vi "Subtract XY (multiple).vi"(8 "error in (no error)":errorcluster, 9 "y":cluster{"X-array":dbl[], "Y-array":dbl[]}, 10 "x":cluster{"X-array":dbl[], "Y-array":dbl[]}, 11 "XY-data":cluster{"X-array":dbl[], "Y-array":dbl[]}[](array[cluster]) {"Y-array" format="%.2p"; "X-array" format="%.2p"}) -> (0 "error out":errorcluster, 3 "XY-data out":cluster{"X-array":dbl[], "Y-array":dbl[]}[](array[cluster]) {"Y-array" format="%.2p"; "X-array" format="%.2p"})   [LabVIEW 2016, in "xy_utilities.lvlib"]
doc: "Subtract <b>x</b>'s x array from the x array of <b>XY-data</b>\nSubtract <b>y</b>'s y array from the y array of <b>XY-data</b>\n\nWire data to the data input to determine the polymorphic instance to use or manually select the instance."
uses:
  xy_utilities.lvlib
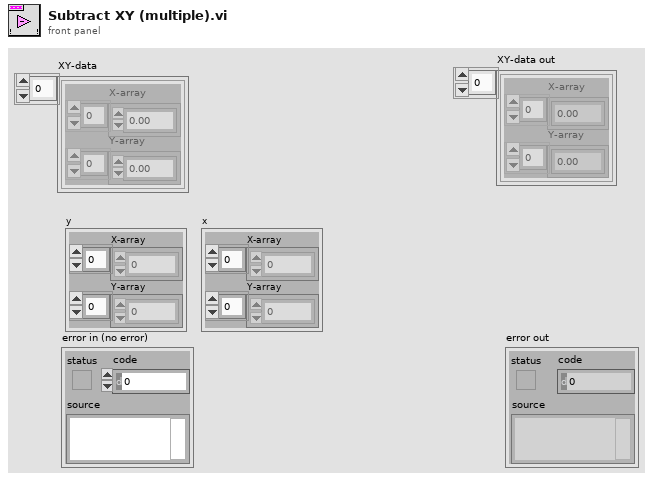
[diagram p1: front panel]
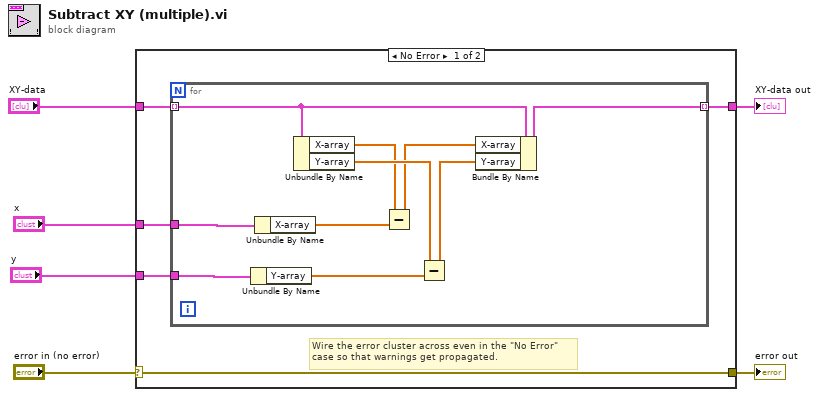
[diagram p0: block diagram]
diagram:
  n1 = case shown="No Error" "error in (no error)" {
    selector: "error in (no error)" -> [w11 w23]
    tunnel: [w11 w23] -> w5
    tunnel: "XY-data" -> [w10 w22]
    tunnel: [w9 w22] -> w3
    tunnel: "y" -> [w8 _]
    tunnel: "x" -> [w7 _]
    frame No Error {
      # "Wire the error cluster across even in the \"No Error\"\ncase so that warnings get propagated."
      n2 = for {
        tunnel: w10 -> [w21] mode=indexing
        tunnel: [w20] -> w9 mode=indexing
        tunnel: w8 -> [w17]
        tunnel: w7 -> [w15]
        n3 = Unbundle By Name(w17) -> ("Y-array"=w16:dbl[])
        n4 = Unbundle By Name(w15) -> ("X-array"=w14:dbl[])
        n5 = Unbundle By Name(w21) -> ("X-array"=w13:dbl[], "Y-array"=w19:dbl[])
        n6 = Subtract(x=w13, y=w14) -> (x-y=w12:dbl[])
        n7 = Subtract(x=w19, y=w16) -> (x-y=w18:dbl[])
        n8 = Bundle By Name(cluster=w21, "X-array"=w12, "Y-array"=w18) -> (w20:cluster{"X-array":dbl[], "Y-array":dbl[]})
      }
    }
    frame Error {
    }
  }
  "error out" <- w5
  "XY-data out" <- w3
